vi "Config.File.Read.vi"(8 "error in":errorcluster, 11 "path":path) -> (0 "error out":errorcluster)   [LabVIEW 2016]
uses:
  Config.Global.vi
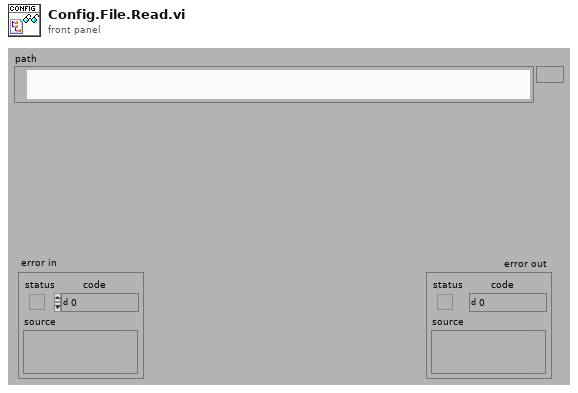
[diagram p1: front panel]
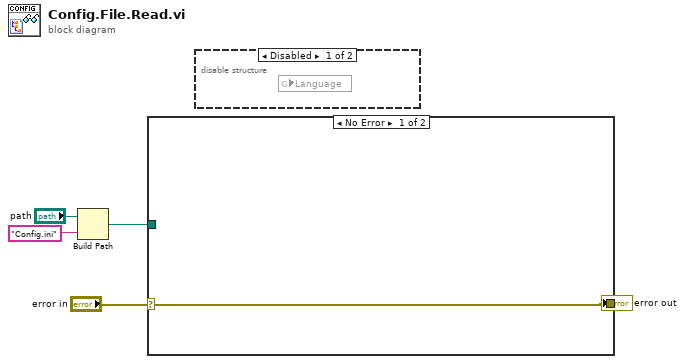
[diagram p0: block diagram]
diagram:
  n1 = Build Path(base path="path", name or relative path="Config.ini") -> (appended path=w1:path)
  n2 = case shown="No Error" "error in" {
    selector: "error in" -> [w6 w7]
    tunnel: [w6 w7] -> w5
    tunnel: w1 -> [_ _]
    frame No Error {
    }
    frame Error {
    }
  }
  "error out" <- w5
  n3 = disable-structure shown="Disabled" {
    frame Disabled {
      n4 = global read "Config.Global.vi" "Language"() -> ()  [unwired: 1 in]
    }
    frame Enabled {
    }
  }
